vi "RAWDATA clean_up.vi"(7 "All?":bool=TRUE, 8 "error in (no error)":errorcluster, 9 "# of scan":i32, 10 "channel":i32[][](array[numeric]), 11 "Detector in":refnum<class "Detector.lvclass">) -> (0 "error out":errorcluster, 1 "channel seq":cluster{"BG":i32[], "Ie":i32[], "I0":i32[]}[](array[cluster]), 3 "Detector out":refnum<class "Detector.lvclass">)   [LabVIEW 2015, in "Detector.lvclass"]
uses:
  Detector.lvclass
panel:
  out "in":i32[][](graph) caption="Data Values"
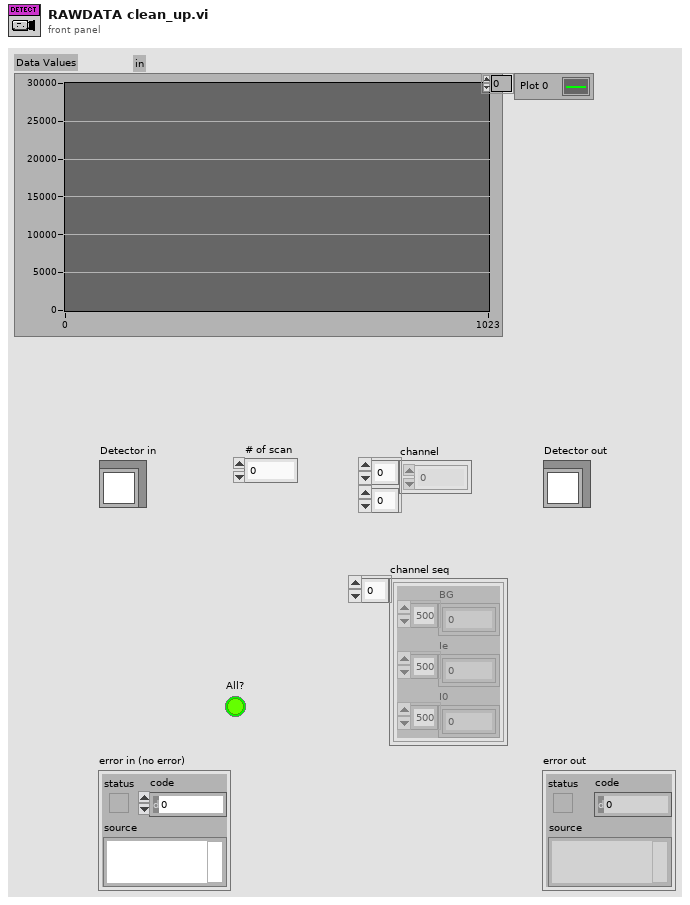
[diagram p1: front panel]
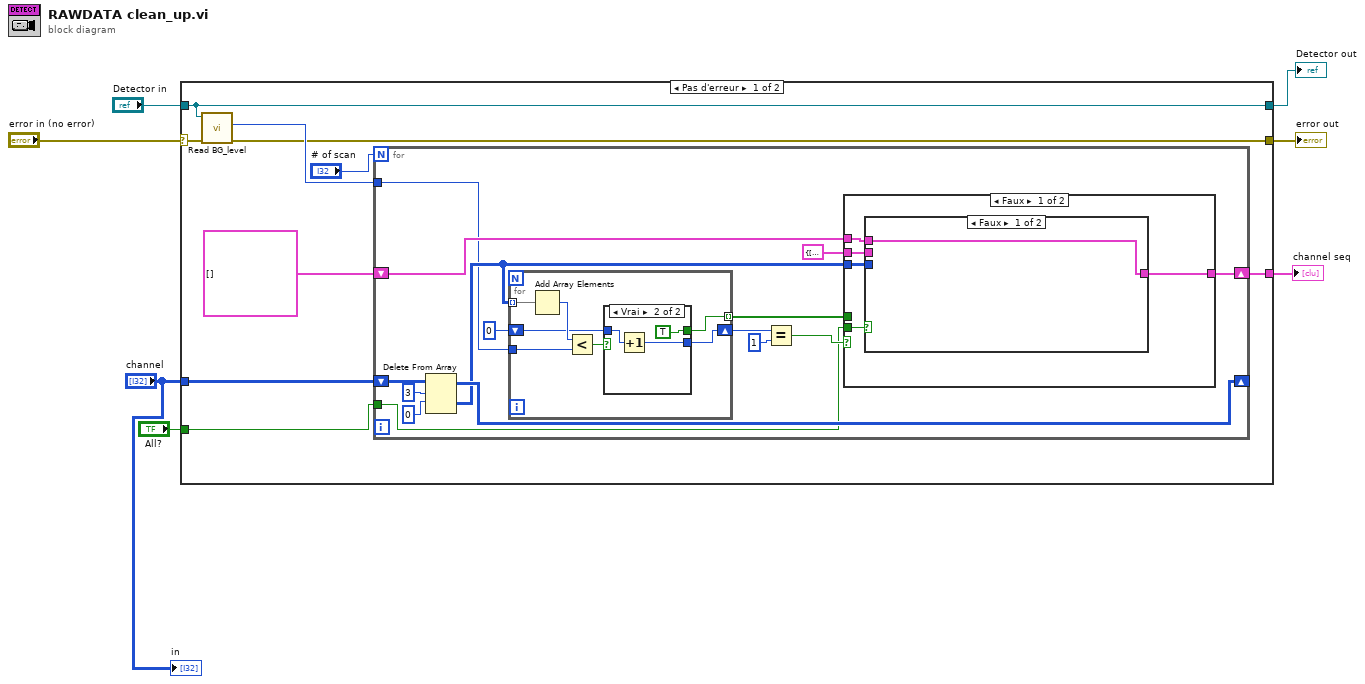
[diagram p0: block diagram]
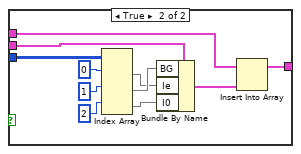
[diagram p2: hidden frame]
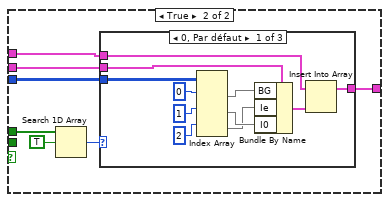
[diagram p3: hidden frame]
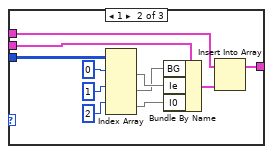
[diagram p4: hidden frame]
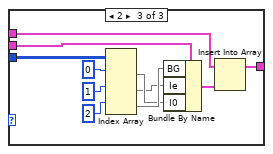
[diagram p5: hidden frame]
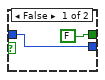
[diagram p6: hidden frame]
diagram:
  n1 = case shown="Pas d'erreur" "error in (no error)" {
    selector: "error in (no error)" -> [w9 w102]
    tunnel: [w8 w102] -> w5
    tunnel: [w11 w101] -> w3
    tunnel: "Detector in" -> [w11 w101]
    tunnel: "All?" -> [w14 _]
    tunnel: "channel" -> [w13 _]
    tunnel: [w12 _] -> w6
    frame No Error {
      n2 = call-dynamic "Read BG_level.vi"("error in (no error)"=w9, "Detector in"=w11) -> ("error out"=w8:errorcluster, "BG_level"=w10:i32)  [unwired: 7 in, 1 out]
      n3 = for {
        N: "# of scan" -> [_]
        shift-right: [w29] -> _
        shift-left: w13 -> [w19]
        shift-right: [w21] -> w12
        shift-left: cluster{"BG":u16[], "Ie":u16[], "I0":u16[]}[] [] -> [w22]
        tunnel: w14 -> [w18]
        tunnel: w10 -> [w17]
        n4 = Delete From Array(array=w19, length=3 ("longueur"), index (row)=0 ("indice (ligne)")) -> (deleted portion=w23:i32[][], array with subset deleted=w29:i32[][])  [unwired: 1 in]
        n5 = for {
          tunnel: w23 -> [w95] mode=indexing
          tunnel: [w92] -> w24 mode=indexing
          shift-right: [w90] -> w27
          shift-left: 0 -> [w91]
          tunnel: w17 -> [w89]
          n6 = Add Array Elements(numeric array=w95) -> (sum=w94:i32)
          n7 = Less?(x=w94, y=w89) -> (x < y?=w93:bool)
          n8 = case shown="Vrai" w93 {
            tunnel: [FALSE TRUE] -> w92
            tunnel: w91 -> [w96 w99]
            tunnel: [w96 w98] -> w90
            frame False {
            }
            frame True {
              n9 = Increment(x=w99) -> (x+1=w98:i32)
            }
          }
        }
        n10 = Equal?(x=w27, y=1) -> (x = y?=w25:bool)
        n11 = case shown="Faux" w25 {
          tunnel: w24 -> [_ w55]
          tunnel: w23 -> [w34 w52]
          tunnel: w22 -> [w36 w51]
          tunnel: [w35 w50] -> w21
          tunnel: cluster{"BG":u16[], "Ie":u16[], "I0":u16[]} {"BG"=[], "Ie"=[], "I0"=[]} ("input cluster") -> [w33 w49]
          tunnel: w18 -> [w32 _]
          frame False {
            n12 = case shown="Faux" w32 {
              tunnel: w36 -> [w37 w41]
              tunnel: [w37 w40] -> w35
              tunnel: w34 -> [_ w39]
              tunnel: w33 -> [_ w38]
              frame False {
              }
              frame True {
                n13 = Index Array(array=w39, index (row) #1=0 ("index (row)"), index (row) #2=1 ("index (row)"), index (row) #3=2 ("index (row)")) -> (element #1=w45:i32[], element #2=w47:i32[], element #3=w46:i32[])  [unwired: 3 in]
                n14 = Bundle By Name(cluster=w38, "BG"=w47, "Ie"=w45, "I0"=w46) -> (w48:cluster{"BG":u16[], "Ie":u16[], "I0":u16[]})
                n15 = Insert Into Array(array=w41, new element=w48) -> (w40:cluster{"BG":u16[], "Ie":u16[], "I0":u16[]}[])  [unwired: 1 in]
              }
            }
          }
          frame True {
            n16 = Search 1D Array(1D array=w55, element=TRUE) -> (index of element=w53:i32)  [unwired: 1 in]
            n17 = case shown="0, Par défaut" w53 {
              tunnel: w52 -> [w63 w74 w85]
              tunnel: w51 -> [w58 w69 w81]
              tunnel: [w57 w68 w79] -> w50
              tunnel: w49 -> [w56 w67 w78]
              frame 0, Default {
                n18 = Index Array(array=w63, index (row) #1=0 ("index (row)"), index (row) #2=1 ("index (row)"), index (row) #3=2 ("index (row)")) -> (element #1=w62:i32[], element #2=w61:i32[], element #3=w60:i32[])  [unwired: 3 in]
                n19 = Bundle By Name(cluster=w56, "BG"=w62, "Ie"=w60, "I0"=w61) -> (w59:cluster{"BG":u16[], "Ie":u16[], "I0":u16[]})
                n20 = Insert Into Array(array=w58, new element=w59) -> (w57:cluster{"BG":u16[], "Ie":u16[], "I0":u16[]}[])  [unwired: 1 in]
              }
              frame 1 {
                n21 = Index Array(array=w74, index (row) #1=0 ("index (row)"), index (row) #2=1 ("index (row)"), index (row) #3=2 ("index (row)")) -> (element #1=w73:i32[], element #2=w71:i32[], element #3=w72:i32[])  [unwired: 3 in]
                n22 = Bundle By Name(cluster=w67, "BG"=w71, "Ie"=w73, "I0"=w72) -> (w70:cluster{"BG":u16[], "Ie":u16[], "I0":u16[]})
                n23 = Insert Into Array(array=w69, new element=w70) -> (w68:cluster{"BG":u16[], "Ie":u16[], "I0":u16[]}[])  [unwired: 1 in]
              }
              frame 2 {
                n24 = Index Array(array=w85, index (row) #1=0 ("index (row)"), index (row) #2=1 ("index (row)"), index (row) #3=2 ("index (row)")) -> (element #1=w83:i32[], element #2=w82:i32[], element #3=w84:i32[])  [unwired: 3 in]
                n25 = Bundle By Name(cluster=w78, "BG"=w84, "Ie"=w82, "I0"=w83) -> (w80:cluster{"BG":u16[], "Ie":u16[], "I0":u16[]})
                n26 = Insert Into Array(array=w81, new element=w80) -> (w79:cluster{"BG":u16[], "Ie":u16[], "I0":u16[]}[])  [unwired: 1 in]
              }
            }
          }
        }
      }
    }
    frame Error {
    }
  }
  "error out" <- w5
  "Detector out" <- w3
  "channel seq" <- w6
  "in" <- "channel"
